vi "Rendevous Kaushik.vi"() -> ()   [LabVIEW 2022 SP3]
panel:
  out "Loop 2":i32
  out "Loop 1":i32
  out "Loop 2 Status":string
  out "Loop 1 Status":string
  in  "error in (no error)":errorcluster
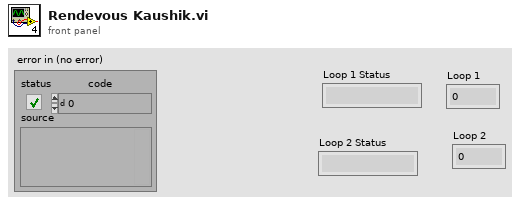
[diagram p1: front panel]
types:
  T1 = typedef "Rendezvous RefNum" = refnum<k1>
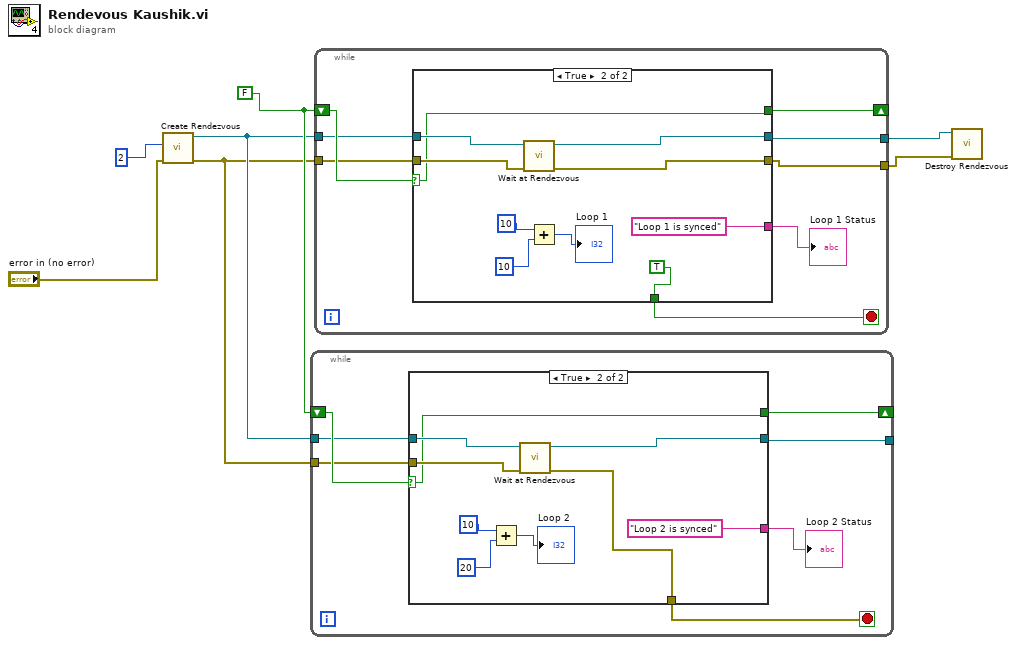
[diagram p0: block diagram]
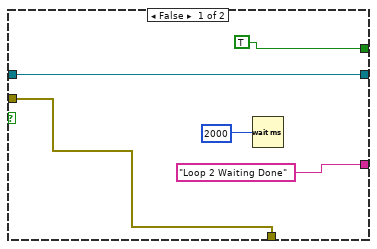
[diagram p2: hidden frame]
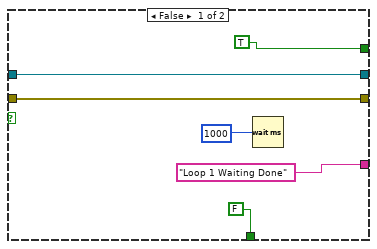
[diagram p3: hidden frame]
diagram:
  w3 = FALSE
  n1 = call <vilib>:"Create Rendezvous.vi"("error in (no error)"="error in (no error)", "size (2)"=2) -> ("error out"=w1:errorcluster, "rendezvous"=w2:T1)  [unwired: 3 in, 1 out]
  n2 = while {
    shift-right: [w10] -> _
    shift-left: w3 -> [w14]
    tunnel: w2 -> [w13]
    tunnel: w1 -> [w12]
    tunnel: [w11] -> _
    stop <- w8 stop-if-true
    n3 = case shown="True" w14 {
      selector: w14 -> [_ w24]
      tunnel: w13 -> [w18 w28]
      tunnel: w12 -> [w15 w27]
      tunnel: [w18 w26] -> w11
      tunnel: [TRUE w24] -> w10
      tunnel: ["Loop 2 Waiting Done" "Loop 2 is synced"] -> w9
      tunnel: [w15 w23] -> w8
      frame False {
        n4 = Wait (ms)(milliseconds to wait=u32 2000) -> ()  [unwired: 1 out]
      }
      frame True {
        n5 = Add(x=10, y=20) -> (x+y=→"Loop 2":i32)
        n6 = call <vilib>:"Wait at Rendezvous.vi"("error in (no error)"=w27, "rendezvous"=w28) -> ("error out"=w23:errorcluster, "rendezvous out"=w26:T1)  [unwired: 3 in, 1 out]
      }
    }
    "Loop 2 Status" <- w9
  }
  n7 = while {
    shift-right: [w31] -> _
    shift-left: w3 -> [w36]
    tunnel: w2 -> [w35]
    tunnel: w1 -> [w34]
    tunnel: [w33] -> w4
    tunnel: [w32] -> w5
    stop <- w29 stop-if-true
    n8 = case shown="True" w36 {
      selector: w36 -> [_ w46]
      tunnel: w35 -> [w40 w52]
      tunnel: w34 -> [w41 w51]
      tunnel: [w41 w49] -> w33
      tunnel: [w40 w50] -> w32
      tunnel: [TRUE w46] -> w31
      tunnel: ["Loop 1 Waiting Done" "Loop 1 is synced"] -> w30
      tunnel: [FALSE TRUE] -> w29
      frame False {
        n9 = Wait (ms)(milliseconds to wait=u32 1000) -> ()  [unwired: 1 out]
      }
      frame True {
        n10 = call <vilib>:"Wait at Rendezvous.vi"("error in (no error)"=w51, "rendezvous"=w52) -> ("error out"=w49:errorcluster, "rendezvous out"=w50:T1)  [unwired: 3 in, 1 out]
        n11 = Add(x=10, y=10) -> (x+y=→"Loop 1":i32)
      }
    }
    "Loop 1 Status" <- w30
  }
  n12 = call <vilib>:"Destroy Rendezvous.vi"("error in (no error)"=w4, "rendezvous"=w5) -> ()  [unwired: 4 in, 2 out]
